vi "ASI Get Product I Ds.vi"(11 "pPIDs":i32) -> (2 "function return":i32, 3 "pPIDs out":i32)   [LabVIEW 2023, in "ASICamera2_no_err.lvlib"]
doc: "ASICAMERA_API int ASIGetProductIDs(int* pPIDs);"
uses:
  ASICamera2_no_err.lvlib
  ASICamera2.dll
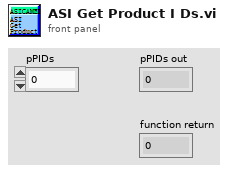
[diagram p1: front panel]
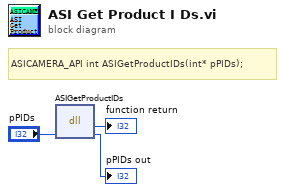
[diagram p0: block diagram]
diagram:
  # "ASICAMERA_API int ASIGetProductIDs(int* pPIDs);"
  n1 = dll-call lib="C:/Users/quantum/Documents/LVDAQ/ConcreteClasses/ConcreteInstrumentClasses/CameraClasses/ZWO_ASI_LV/Labview_ASI_demo_64bit_221128/user.lib/ASICamera2_no_err/ASICamera2.*" fn="ASIGetProductIDs"("pPIDs"="pPIDs") -> (→"function return":i32, "pPIDs"=→"pPIDs out":i32)  [unwired: 3 in, 2 out]
